vi "Write Interface Configs.vi"(8 "error in (no error)":errorcluster, 10 "Device Ref in":T2 format="%.0x", 11 "Refnum in":T1) -> (0 "error out":errorcluster, 2 "Item Ref out":T2 format="%.0x", 3 "Refnum out":T1)   [LabVIEW 2021, in "Modbus Master System Explorer.lvlib"]
uses:
  Modbus Master System Explorer.lvlib
  <vilib>/NI VeriStand/Custom Device API/Custom Device Item Ref.ctl
  <vilib>/Utility/config.llb/Config Data RefNum.ctl
  <vilib>/Utility/config.llb/Write Key (String).vi
  <vilib>/Utility/config.llb/Write Key (U32).vi
  <vilib>/Utility/config.llb/Write Key (I32).vi
  <vilib>/Utility/config.llb/NI_LVConfig.lvlib
  <vilib>/NI VeriStand/Custom Device API/Custom Device API.lvlib
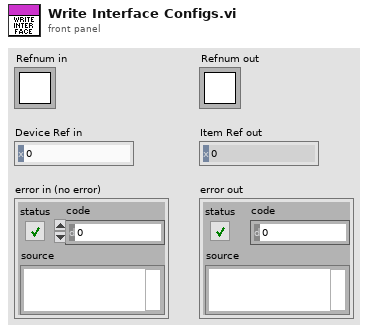
[diagram p1: front panel]
types:
  T1 = typedef "NI_LVConfig.lvlib/Config Data RefNum.ctl" = refnum<k1>
  T2 = typedef "Custom Device API.lvlib/Custom Device Item Ref.ctl" = u64
  T3 = typedef "Modbus Master Shared.lvlib/Interface Type.ctl" = enum16{"TCP Master", "Serial Master", "TCP Slave", "Serial Slave"}
  T4 = typedef "Modbus Master Shared.lvlib/Write Mode.ctl" = enum16{"Value Change", "Interval"}
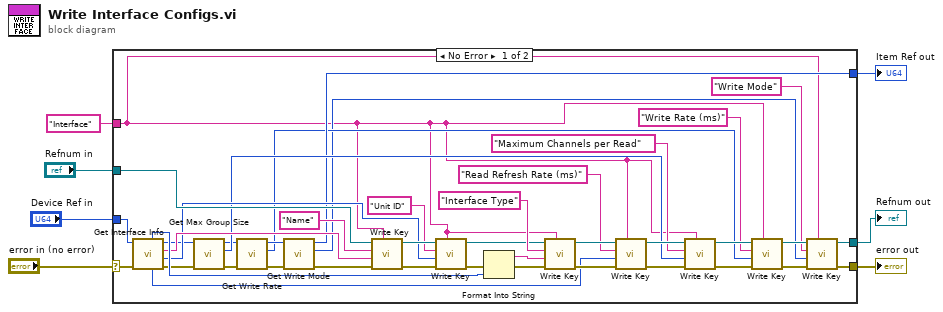
[diagram p0: block diagram]
diagram:
  n1 = case shown="No Error" "error in (no error)" {
    selector: "error in (no error)" -> [w43 w50]
    tunnel: [w15 w52] -> w7
    tunnel: [w20 w50] -> w6
    tunnel: [w19 w51] -> w5
    tunnel: "Interface" ("section") -> [w10 _]
    tunnel: "Device Ref in" -> [w42 w52]
    tunnel: "Refnum in" -> [w41 w51]
    frame No Error {
      n2 = call "Get Interface Info.vi"("error in (no error)"=w43, "Device Item Ref in"=w42) -> ("error out"=w25:errorcluster, "Unit ID"=w36:u16, "Name"=w39:string, "Item Ref out"=w27:T2, "Refresh Rate"=w28:i32, "Interface Type"=w48:T3)  [unwired: 4 in]
      n3 = call "Get Max Group Size.vi"("error in (no error)"=w25, "Item Ref in"=w27) -> ("error out"=w14:errorcluster, "Value"=w26:i32, "Item Ref out"=w18:T2)  [unwired: 7 in]
      n4 = call "Get Write Rate.vi"("error in (no error)"=w14, "Item Ref in"=w18) -> ("error out"=w16:errorcluster, "Value"=w12:i32, "Item Ref out"=w17:T2)  [unwired: 7 in]
      n5 = call "Get Write Mode.vi"("error in (no error)"=w16, "Item Ref in"=w17) -> ("error out"=w13:errorcluster, "Write Mode"=w11:T4, "Item Ref out"=w15:T2)  [unwired: 7 in]
      n6 = call-poly <vilib>:"Write Key.vi"("section"=w10, "error in (no error)"=w13, "value"=w39, "key"="Name", "refnum"=w41) -> ("error out"=w38:errorcluster, "refnum out"=w37:T1)  [unwired: 4 in, 1 out]
      n7 = call-poly <vilib>:"Write Key.vi"("section"=w10, "error in (no error)"=w38, "value"=w36, "key"="Unit ID", "refnum"=w37) -> ("error out"=w46:errorcluster, "refnum out"=w44:T1)  [unwired: 4 in, 1 out]
      n8 = Format Into String(error in=w46, w48) -> (resulting string=w49:string, error out=w47:errorcluster)  [unwired: 2 in]
      n9 = call-poly <vilib>:"Write Key.vi"("section"=w10, "error in (no error)"=w47, "value"=w49, "key"="Interface Type", "refnum"=w44) -> ("error out"=w34:errorcluster, "refnum out"=w33:T1)  [unwired: 4 in, 1 out]
      n10 = call-poly <vilib>:"Write Key.vi"("section"=w10, "error in (no error)"=w34, "value"=w28, "key"="Read Refresh Rate (ms)", "refnum"=w33) -> ("error out"=w31:errorcluster, "refnum out"=w30:T1)  [unwired: 4 in, 1 out]
      n11 = call-poly <vilib>:"Write Key.vi"("section"=w10, "error in (no error)"=w31, "value"=w26, "key"="Maximum Channels per Read", "refnum"=w30) -> ("error out"=w24:errorcluster, "refnum out"=w23:T1)  [unwired: 4 in, 1 out]
      n12 = call-poly <vilib>:"Write Key.vi"("section"=w10, "error in (no error)"=w24, "value"=w12, "key"="Write Rate (ms)", "refnum"=w23) -> ("error out"=w21:errorcluster, "refnum out"=w22:T1)  [unwired: 4 in, 1 out]
      n13 = call-poly <vilib>:"Write Key.vi"("section"=w10, "error in (no error)"=w21, "value"=w11, "key"="Write Mode", "refnum"=w22) -> ("error out"=w20:errorcluster, "refnum out"=w19:T1)  [unwired: 4 in, 1 out]
    }
    frame Error {
    }
  }
  "Item Ref out" <- w7
  "error out" <- w6
  "Refnum out" <- w5
